vi "Cleanup.vi"(8 "error in (no error)":errorcluster, 11 "GodotServer in":refnum<class "GodotServer.lvclass">) -> (0 "error out":errorcluster)   [LabVIEW 2020, in "GodotLV.lvlib" / "GodotServer.lvclass"]
doc: "Closes down and releases all resources for the server."
uses:
  GodotServer.lvclass
  GodotServer.lvclass/GodotServer.ctl
  <vilib>/IlluminatedG/IG WebSocket Stream/Stream-Websocket/Websocket Server/Websocket Server.lvclass
  <vilib>/IlluminatedG/IG HTTP Server/HTTP Server/Server/Server.lvclass
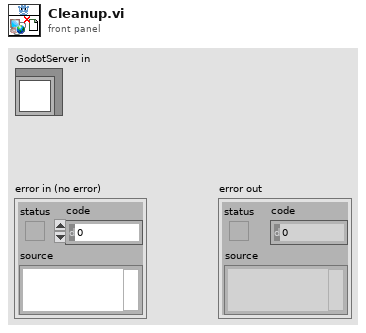
[diagram p1: front panel]
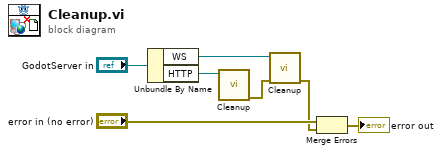
[diagram p0: block diagram]
diagram:
  n1 = Unbundle By Name("GodotServer in") -> ("WS"=w3:refnum<class "Websocket Server.lvclass">, "HTTP"=w5:refnum<class "Server.lvclass">)
  n2 = call <vilib>:"Cleanup.vi"("Server in"=w5) -> ("error out"=w2:errorcluster)  [unwired: 10 in]
  n3 = call-dynamic <vilib>:"Cleanup.vi"("error in (no error)"=w2, "Websocket Server in"=w3) -> ("error out"=w1:errorcluster)  [unwired: 9 in]
  n4 = Merge Errors("error in (no error)", w1) -> (→"error out":errorcluster)
